vi "Print HTML Report.vi"(0 "report in":refnum<class "NI_report.lvclass">, 11 "error in (no error)":errorcluster) -> (4 "report out":refnum<class "NI_report.lvclass">, 15 "error out":errorcluster)   [LabVIEW 2015, in "NI_ReportGenerationCore.lvlib"]
doc: "This VI prints an HTML Report using Internet Explorer."
uses:
  <vilib>/Utility/NIReport.llb/NI_ReportGenerationCore.lvlib
  <vilib>/Utility/NIReport.llb/NI_report.lvclass
  <vilib>/registry/registry.llb/Registry RtKey.ctl
  <vilib>/registry/registry.llb/Read Registry Value Simple STR.vi
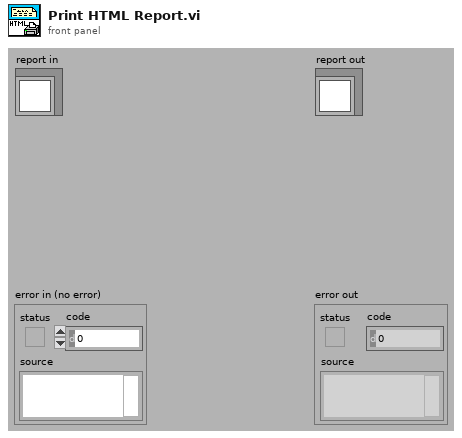
[diagram p1: front panel]
types:
  T1 = typedef "Registry RtKey.ctl" = enum32{"HKEY_CLASSES_ROOT", "HKEY_CURRENT_USER", "HKEY_LOCAL_MACHINE", "HKEY_USERS", "HKEY_PERFORMANCE_DATA", "HKEY_CURRENT_CONFIG", "HKEY_DYN_DATA"}
  T2 = enum32{"KEY_QUERY_VALUE", "KEY_SET_VALUE", "KEY_CREATE_SUB_KEY", "KEY_ENUMERATE_SUB_KEYS", "KEY_NOTIFY", "KEY_CREATE_LINK", "KEY_READ", "KEY_WRITE", "KEY_ALL_ACCESS", "KEY_READ | KEY_WRITE"}
  T3 = typedef "Registry refnum.ctl" = refnum<k1>
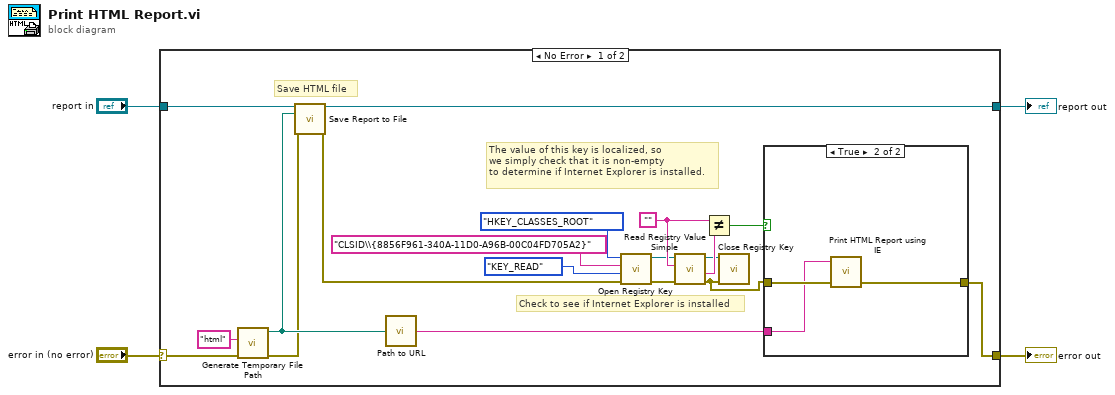
[diagram p0: block diagram]
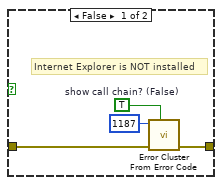
[diagram p2: hidden frame]
diagram:
  n1 = case shown="No Error" "error in (no error)" {
    selector: "error in (no error)" -> [w6 w31]
    tunnel: "report in" -> [w11 w32]
    tunnel: [w10 w32] -> w2
    tunnel: [w9 w31] -> w1
    frame No Error {
      w22 = ""
      # "The value of this key is localized, so\nwe simply check that it is non-empty\nto determine if Internet Explorer is installed."
      # "Check to see if Internet Explorer is installed"
      # "Save HTML file"
      n2 = call <vilib>:"Generate Temporary File Path.vi"("error in (no error)"=w6, "Temporary File Extension (tmp)"="html") -> ("error out"=w5:errorcluster, "Unique Temporary File Path"=w7:path)  [unwired: 8 out]
      n3 = call-dynamic "Save Report to File.vi"("report in"=w11, "report file path"=w7, "error in (no error)"=w5) -> ("report out"=w10:refnum<class "NI_report.lvclass">, "error out"=w21:errorcluster)  [unwired: 11 in]
      n4 = call <vilib>:"Path to URL.vi"("path"=w7) -> ("url"=w12:string)
      n5 = call <vilib>:"Open Registry Key.vi"("error in (no error)"=w21, "security access mask (KEY_READ | KEY_WRITE)"=T2."KEY_READ", "subkey"="CLSID\\{8856F961-340A-11D0-A96B-00C04FD705A2}", "root key (HKEY_LOCAL_MACHINE)"=Registry_RtKey."HKEY_CLASSES_ROOT") -> ("error out"=w17:errorcluster, "refnum out"=w19:T3)  [unwired: 6 out]
      n6 = call-poly <vilib>:"Read Registry Value Simple.vi"("error in (no error)"=w17, "value"=w22, "refnum"=w19) -> ("error out"=w23:errorcluster, "String/Binary data"=w14:string, "refnum out"=w13:T3)  [unwired: 1 in, 3 out]
      n7 = Not Equal?(x=w22, y=w14) -> (x != y?=w20:bool)
      n8 = call <vilib>:"Close Registry Key.vi"("error in (no error)"=w23, "refnum"=w13) -> ()  [unwired: 6 out]
      n9 = case shown="True" w20 {
        tunnel: [w25 w28] -> w9
        tunnel: w23 -> [w26 w30]
        tunnel: w12 -> [_ w29]
        frame False {
          w24 = TRUE  # show call chain? (False)
          # "Internet Explorer is NOT installed"
          n10 = call <vilib>:"Error Cluster From Error Code.vi"("show call chain? (False)"=w24, "error in (no error)"=w26, "error code (0)"=1187) -> ("error out"=w25:errorcluster)  [unwired: 6 out]
        }
        frame True {
          n11 = call <vilib>:"Print HTML Report using IE.vi"("error in (no error)"=w30, "path to HTML"=w29) -> ("error out"=w28:errorcluster)  [unwired: 3 out]
        }
      }
    }
    frame Error {
    }
  }
  "report out" <- w2
  "error out" <- w1
